vi "Init.vi"(8 "error in (no error)":errorcluster, 11 "Data in":refnum<class "Alias Bus.lvclass">) -> (0 "error out":errorcluster, 3 "Data out":refnum<class "Alias Bus.lvclass">)   [LabVIEW 2021, in "Alias Bus.lvclass"]
doc: "Abstract Data Classes 2.1.1.12\nTim Streeter - TSA\nCopyright (c) 2024, TSA"
uses:
  Alias Bus.lvclass
  C:/TSA/Omni-Bus/Source/Omni-Bus/Bus Access/Bus_Access.lvclass
  Alias Bus.lvclass/Alias Bus.ctl
  Omni-Bus/Bus Access/Bus_Access.lvclass/Bus_Access.ctl
  Omni-Bus/Bus Access/Properties/Read Tags.vi
  Omni-Bus/Bus Access/Properties/Read Values.vi
  Properties/Read Buses.vi
  Properties/Read Map.vi
  Properties/Read Keep Original.vi
  Properties/Write Buses.vi
  Omni-Bus/Bus Access/Properties/Write Tags.vi
  Omni-Bus/Bus Access/Properties/Write Values.vi
  Omni-Bus/Bus Access/Bus_Access.lvclass
  <vilib>/TSA/Abstract Data Classes/Abs_Types/Type/Abs_Type.lvclass
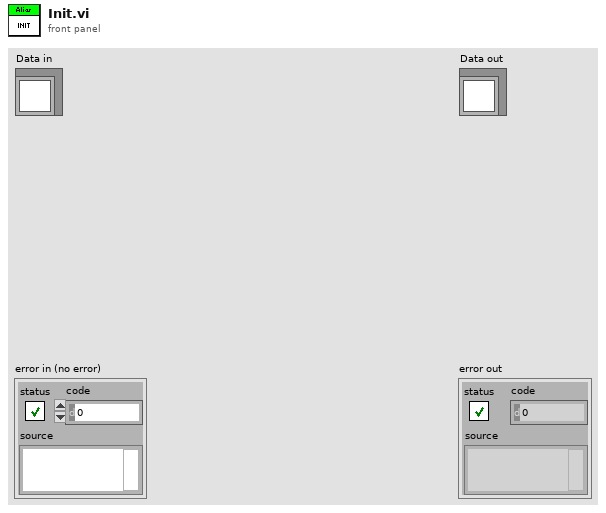
[diagram p1: front panel]
types:
  T1 = typedef "Alias Bus.lvclass/Remap Type.ctl" = map{string, string}
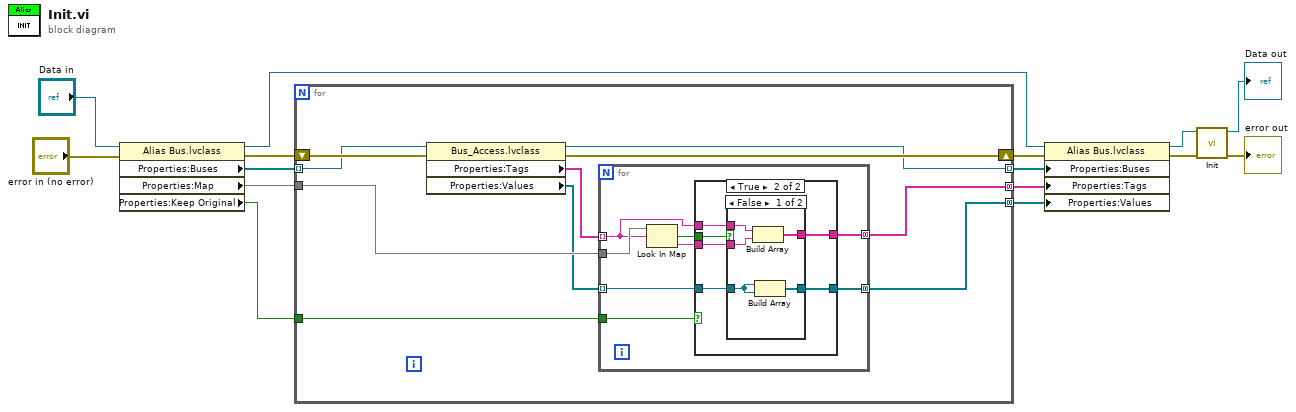
[diagram p0: block diagram]
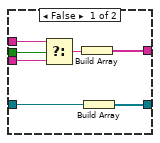
[diagram p2: hidden frame]
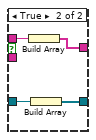
[diagram p3: hidden frame]
diagram:
  n1 = property class="Alias Bus.lvclass"(reference="Data in", error in="error in (no error)") -> (reference out=w8:refnum<class "Alias Bus.lvclass">, error out=w12:errorcluster, "Properties:Buses"=w13:refnum<class "Bus_Access.lvclass">[], "Properties:Map"=w11:T1, "Properties:Keep Original"=w5:bool)
  n2 = for {
    tunnel: w13 -> [w22] mode=indexing
    shift-right: [w21] -> w10
    shift-left: w12 -> [w23]
    tunnel: w11 -> [w25]
    tunnel: [w20] -> w9 mode=indexing
    tunnel: [w19] -> w7 mode=concatenating
    tunnel: [w17] -> w6 mode=concatenating
    tunnel: w5 -> [w16]
    n3 = property class="Bus_Access.lvclass"(reference=w22, error in=w23) -> (reference out=w20:refnum<class "Bus_Access.lvclass">, error out=w21:errorcluster, "Properties:Tags"=w24:string[], "Properties:Values"=w18:refnum<class "Abs_Type.lvclass">[])
    n4 = for {
      tunnel: w25 -> [w33]
      tunnel: w24 -> [w30] mode=indexing
      tunnel: [w28] -> w19 mode=concatenating
      tunnel: w18 -> [w29] mode=indexing
      tunnel: [w27] -> w17 mode=concatenating
      tunnel: w16 -> [w26]
      n5 = Look In Map(map=w33, key=w30) -> (key not found?=w31:bool, value=w32:string)  [unwired: 1 in]
      n6 = case shown="True" w26 {
        tunnel: w32 -> [w40 w45]
        tunnel: w31 -> [w39 w46]
        tunnel: w30 -> [w38 w44]
        tunnel: [w34 w43] -> w28
        tunnel: w29 -> [w36 w42]
        tunnel: [w35 w41] -> w27
        frame False {
          n7 = Select(t=w38, s=w39, f=w40) -> (s? t:f=w37:string)
          n8 = Build Array(w37) -> (w34:string[])
          n9 = Build Array(w36) -> (w35:refnum<class "Abs_Type.lvclass">[])
        }
        frame True {
          n10 = case shown="False" w46 {
            tunnel: w45 -> [w50 _]
            tunnel: w44 -> [w51 w55]
            tunnel: [w49 w54] -> w43
            tunnel: w42 -> [w48 w53]
            tunnel: [w47 w52] -> w41
            frame False {
              n11 = Build Array(w51, w50) -> (w49:string[])
              n12 = Build Array(w48, w48) -> (w47:refnum<class "Abs_Type.lvclass">[])
            }
            frame True {
              n13 = Build Array(w55) -> (w54:string[])
              n14 = Build Array(w53) -> (w52:refnum<class "Abs_Type.lvclass">[])
            }
          }
        }
      }
    }
  }
  n15 = property class="Alias Bus.lvclass"(reference=w8, error in=w10, "Properties:Buses"=w9, "Properties:Tags"=w7, "Properties:Values"=w6) -> (reference out=w2:refnum<class "Alias Bus.lvclass">, error out=w4:errorcluster)
  n16 = call-parent "Init.vi"("error in (no error)"=w4, "Data in"=w2) -> ("error out"=→"error out":errorcluster, "Data out"=→"Data out":refnum<class "Alias Bus.lvclass">)  [unwired: 8 in]
